vi "Remove driveletter on 1 axis system.vi"(4 "Config in":T2(array[cluster])) -> (1 "Config out":T2(array[cluster]))   [LabVIEW 2019]
uses:
  Axis enum.ctl
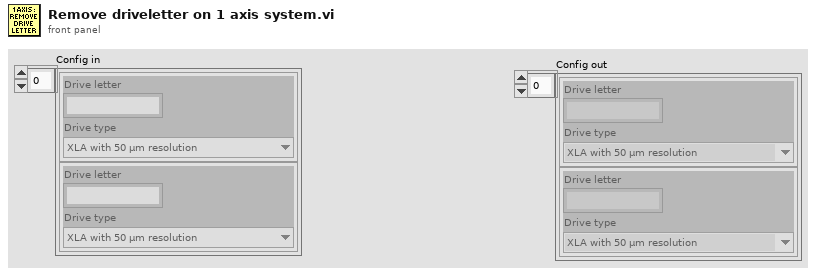
[diagram p1: front panel]
types:
  T1 = typedef "Axis enum.ctl" = enum16{"XLA with 50 µm resolution", "XLA with 10 µm resolution", "XLA with 1250 nm resolution", "XLA with 312 nm resolution", "XLA with 78 nm resolution", "XLS with 1250 nm resolution", "XLS with 312 nm resolution", "XLS with 78nm resolution", "XLS with 5nm resolution", "XLS with 1 nm resolution", "XRT-A with 109 µrad resolution", "XRT-U-30 with 109 µrad resolution", "XRT-U-30 with 49 µrad resolution", "XRT-U-30 with 19 µrad resolution", "XRT-U-30 with 3 µrad resolution", "XRT-U-40 with 109 µrad resolution", "XRT-U 40 with 49 µrad resolution", "XRT-U-40 with 19 µrad resolution", "XRT-U-40 with 3 µrad resolution", "XRT-U-60 with 109 µrad resolution", "XRT-U-60 with 49 µrad resolution", "XRT-U-60 with 19 µrad resolution", "XRT-U-60 with 3 µrad resolution"}
  T2 = cluster{"Drive letter":string, "Drive type":T1}[]
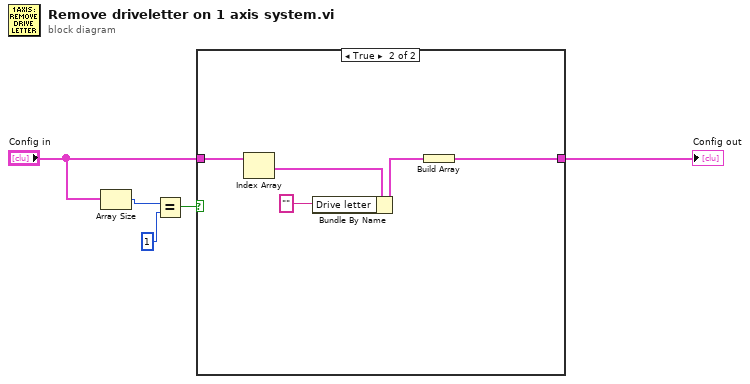
[diagram p0: block diagram]
diagram:
  n1 = Array Size(array="Config in") -> (size(s)=w5:i32)
  n2 = Equal?(x=w5, y=1) -> (x = y?=w3:bool)
  n3 = case shown="True" w3 {
    tunnel: [w6 w7] -> w1
    tunnel: "Config in" -> [w6 w11]
    frame False {
    }
    frame True {
      n4 = Index Array(array=w11) -> (element=w10:cluster{"Drive letter":string, "Drive type":T1})  [unwired: 1 in]
      n5 = Bundle By Name(cluster=w10, "Drive letter"="" ("Letter")) -> (w8:cluster{"Drive letter":string, "Drive type":T1})
      n6 = Build Array(w8) -> (w7:T2)
    }
  }
  "Config out" <- w1
